vi "_List Example VIs.vi"(11 "root":path) -> (3 "Array":path[](array[path]))   [LabVIEW 2017, in "csmdoc.lvlib"]
uses:
  csmdoc.lvlib
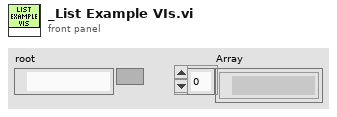
[diagram p1: front panel]
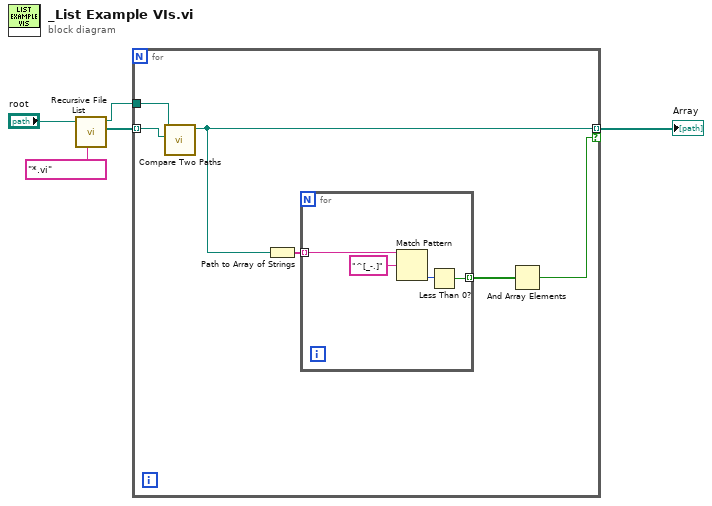
[diagram p0: block diagram]
diagram:
  n1 = call <vilib>:"Recursive File List.vi"("pattern"="*.vi", "Folder Path"="root") -> ("All Files in Dir"=w3:path[], "dup Folder Path"=w2:path)  [unwired: 5 in, 3 out]
  n2 = for {
    tunnel: w3 -> [w11] mode=indexing
    tunnel: [w8] -> w1 mode=indexing if=w6
    tunnel: w2 -> [w10]
    n3 = call <vilib>:"Compare Two Paths.vi"("Path 2"=w11, "Path 1"=w10) -> ("Relative Path from 1 to 2"=w8:path)  [unwired: 6 in, 3 out]
    n4 = Path to Array of Strings(0:w8) -> (2:w9:string[])  [unwired: 1 out]
    n5 = for {
      tunnel: w9 -> [w15] mode=indexing
      tunnel: [w12] -> w7 mode=indexing
      n6 = Match Pattern(string=w15, regular expression="^[_-.]") -> (offset past match=w13:i32)  [unwired: 1 in, 3 out]
      n7 = Less Than 0?(x=w13) -> (x < 0?=w12:bool)
    }
    n8 = And Array Elements(Boolean array=w7) -> (logical AND=w6:bool)
  }
  "Array" <- w1
